vi "Close kinect systems Dani.vi"(8 "error in (no error)":errorcluster) -> (0 "error out":errorcluster)   [LabVIEW 2015]
uses:
  Controls/Led Control.ctl
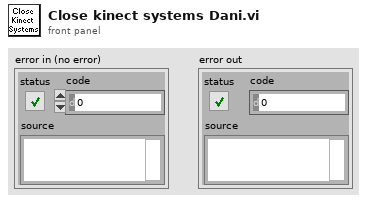
[diagram p1: front panel]
types:
  T1 = typedef "Led Control.ctl" = enum32{"LED_OFF", "LED_GREEN", "LED_RED", "LED_YELLOW", "LED_BLINK_GREEN", "LED_BLINK_GREEN2", "LED_BLINK_RED_YELLOW"}
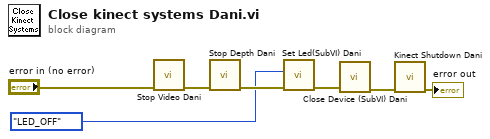
[diagram p0: block diagram]
diagram:
  n1 = call "Stop Video Dani.vi"("error in (no error)"="error in (no error)") -> ("error out"=w1:errorcluster)  [unwired: 10 in]
  n2 = call "Stop Depth Dani.vi"("error in (no error)"=w1) -> ("error out"=w7:errorcluster)  [unwired: 10 in]
  n3 = call "Set Led(SubVI) Dani.vi"("error in (no error)"=w7, "Led Option"=Led_Control."LED_OFF") -> ("error out"=w6:errorcluster)  [unwired: 9 in]
  n4 = call "Close Device (SubVI) Dani.vi"("error in (no error)"=w6) -> ("error out"=w4:errorcluster)  [unwired: 10 in]
  n5 = call "Kinect Shutdown Dani.vi"("error in (no error)"=w4) -> ("error out"=→"error out":errorcluster)  [unwired: 10 in]
